vi "RT Driver VI.vi"(7 "Operation":T1(ring), 11 "Device Reference in":u64 format="%.0x") -> (0 "Error Code":i32)   [LabVIEW 2026, in "SystemMonitor Engine.lvlib"]
uses:
  SystemMonitor Engine.lvlib
  VS Custom Device API/NIVS Custom Device API.lvclass
  C:/SysMon1/SystemMonitor Custom Device/Auto Generated/Engine/VS Custom Device API/NIVS Custom Device API.lvclass
  C:/Program Files/NI/LVAddons/nivscustomdeviceexpress/1/Targets/win64/user.lib/Custom Device Interfaces_v1.lvlibp/CustomDeviceAPI/Custom Device API.lvclass
  <userlib>/Custom Device Interfaces_v1.lvlibp/Utility/Custom Device Utility.lvclass
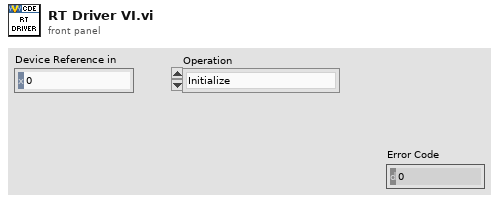
[diagram p1: front panel]
types:
  T1 = enum16{"Initialize", "Start", "Read Data from HW", "Write Data to HW", "Close"}
  T2 = cluster{"Custom Device Utility":refnum<class "Custom Device Utility.lvclass">}
  T3 = cluster{"Name":string, "PPL Path":path, "Instance Name":string, "Compiled Settings":variant}
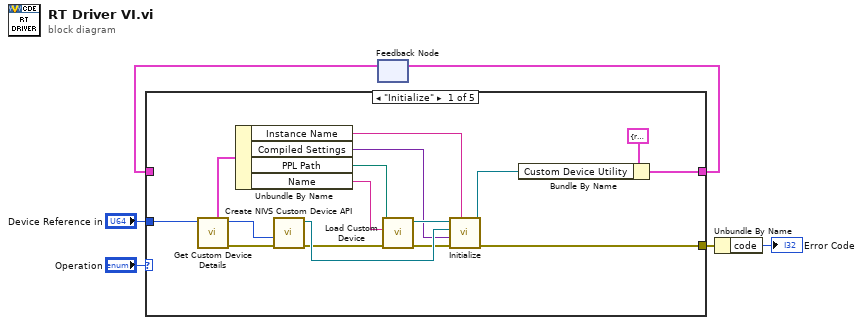
[diagram p0: block diagram]
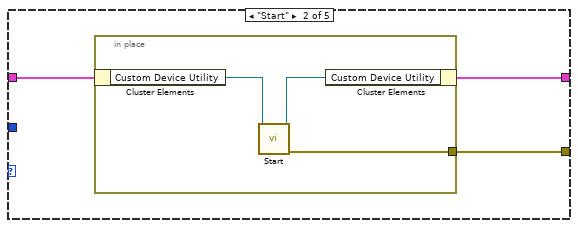
[diagram p2: hidden frame]
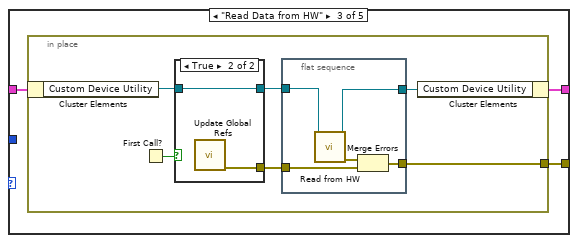
[diagram p3: hidden frame]
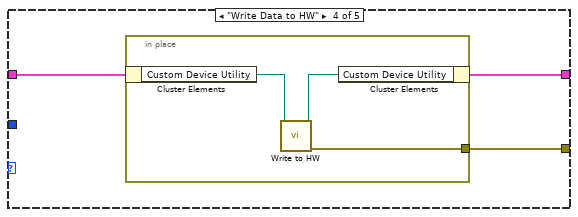
[diagram p5: hidden frame]
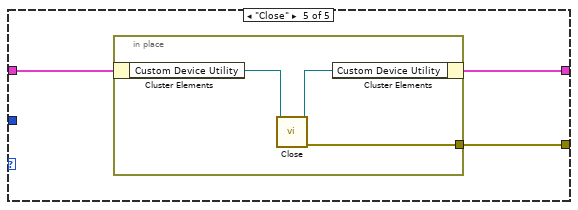
[diagram p6: hidden frame]
diagram:
  n1 = feedback #1() -> (w3:T2)  [unwired: 1 in]
  n2 = case shown="\"Initialize\"" "Operation" {
    tunnel: [w18 w24 w29 w46 w52] -> w4
    tunnel: w3 -> [_ w23 w30 w47 w53]
    tunnel: "Device Reference in" -> [w16 _ _ _ _]
    tunnel: [w22 w25 w31 w48 w54] -> w6
    frame "Initialize" {
      n3 = call "Get Custom Device Details.vi"("Device Reference in"=w16) -> ("error out"=w15:errorcluster, "Data Reference out"=w14:u64, "Custom Device Details"=w13:T3)  [unwired: 8 in]
      n4 = Unbundle By Name(w13) -> ("Instance Name"=w12:string, "Compiled Settings"=w11:variant, "PPL Path"=w8:path, "Name"=w7:string)
      n5 = call "Create NIVS Custom Device API.vi"("error in"=w15, "Custom Device Item Ref"=w14) -> ("error out"=w10:errorcluster, "NIVS Custom Device API out"=w17:refnum<class "NIVS Custom Device API.lvclass">)  [unwired: 8 in]
      n6 = call <userlib>:"Load Custom Device.vi"("error in"=w10, "Custom Device Name"=w7, "Path"=w8) -> ("error out"=w9:errorcluster, "Custom Device out"=w21:refnum<class "Custom Device.lvclass">)  [unwired: 7 in]
      n7 = call <userlib>:"Initialize.vi"("Custom Device in"=w21, "Custom Device Name"=w12, "error in"=w9, "Compiled Settings"=w11, "Custom Device API in"=w17) -> ("error out"=w22:errorcluster, "Custom Device Utility out"=w19:refnum<class "Custom Device Utility.lvclass">)  [unwired: 5 in]
      n8 = Bundle By Name(cluster=T2 {"Custom Device Utility"=refnum}, "Custom Device Utility"=w19) -> (w18:T2)
    }
    frame "Start" {
      n9 = in-place {
        in-place-border: [w28] -> w25
        n10 = in-place-cluster #2(w23) -> ("Custom Device Utility"=w27:refnum<class "Custom Device Utility.lvclass">)
        n11 = call <userlib>:"Start.vi"("Custom Device Utility in"=w27) -> ("error out"=w28:errorcluster, "Custom Device Utility out"=w26:refnum<class "Custom Device Utility.lvclass">)  [unwired: 9 in]
        n12 = in-place-cluster #2("Custom Device Utility"=w26) -> (w24:T2)
      }
    }
    frame "Read Data from HW" {
      n13 = in-place {
        in-place-border: [w37] -> w31
        n14 = in-place-cluster #3(w30) -> ("Custom Device Utility"=w34:refnum<class "Custom Device Utility.lvclass">)
        n15 = First Call?() -> (First Call?: T/F=w35:bool)
        n16 = case shown="True" w35 {
          tunnel: [_ w45] -> w36
          tunnel: w34 -> [w43 w44]
          tunnel: [w43 w44] -> w33
          frame False {
          }
          frame True {
            n17 = call "Update Global Refs.vi"() -> ("error out"=w45:errorcluster)  [unwired: 11 in]
          }
        }
        n18 = flat-sequence {
          tunnel: [w41] -> w37
          tunnel: w36 -> [w40]
          tunnel: w33 -> [w38]
          tunnel: [w39] -> w32
          frame #0 {
            n19 = call <userlib>:"Read from HW.vi"("Custom Device Utility in"=w38) -> ("error out"=w42:errorcluster, "Custom Device Utility out"=w39:refnum<class "Custom Device Utility.lvclass">)  [unwired: 9 in]
            n20 = Merge Errors(w42, w40) -> (w41:errorcluster)
          }
        }
        n21 = in-place-cluster #3("Custom Device Utility"=w32) -> (w29:T2)
      }
    }
    frame "Write Data to HW" {
      n22 = in-place {
        in-place-border: [w51] -> w48
        n23 = in-place-cluster #4(w47) -> ("Custom Device Utility"=w50:refnum<class "Custom Device Utility.lvclass">)
        n24 = call <userlib>:"Write to HW.vi"("Custom Device Utility in"=w50) -> ("error out"=w51:errorcluster, "Custom Device Utility out"=w49:refnum<class "Custom Device Utility.lvclass">)  [unwired: 9 in]
        n25 = in-place-cluster #4("Custom Device Utility"=w49) -> (w46:T2)
      }
    }
    frame "Close" {
      n26 = in-place {
        in-place-border: [w57] -> w54
        n27 = in-place-cluster #5(w53) -> ("Custom Device Utility"=w56:refnum<class "Custom Device Utility.lvclass">)
        n28 = call <userlib>:"Close.vi"("Custom Device Utility in"=w56) -> ("error out"=w57:errorcluster, "Custom Device Utility out"=w55:refnum<class "Custom Device Utility.lvclass">)  [unwired: 9 in]
        n29 = in-place-cluster #5("Custom Device Utility"=w55) -> (w52:T2)
      }
    }
  }
  n30 = feedback-in #1(w4) -> ()
  n31 = Unbundle By Name(w6) -> ("code"=→"Error Code":i32)
